vi "View.vi"(0 "object in":refnum<class "DataType.lvclass">, 2 "Requirements":T2, 5 "error in (no error)":errorcluster) -> (14 "object out":refnum<class "DataType.lvclass">, 16 "Message":T1, 19 "error out":errorcluster)   [LabVIEW 2024, in "DataType.lvclass"]
uses:
  DataType.lvclass
  Support/Type Def/Requirements.ctl
  Support/Type Def/File Type.ctl
  Support/Type Def/Message.ctl
  DataType.lvclass/DataType.ctl
panel:
  # "Connector Pane"
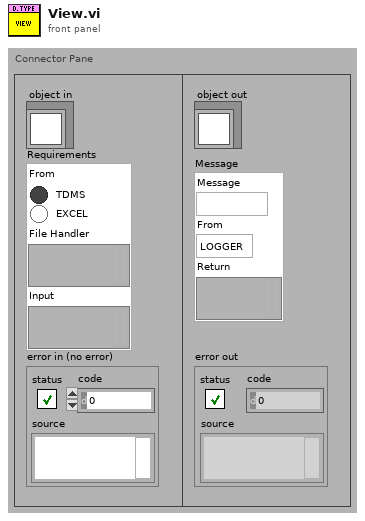
[diagram p1: front panel]
types:
  T1 = typedef "Message.ctl" = cluster{"Message":string, "From":enum16{"LOGGER", "VIEWER"}, "Return":variant}
  T2 = typedef "Requirements.ctl" = cluster{"From":T3, "File Handler":variant, "Input":variant}
  T3 = typedef "File Type.ctl" = enum32{"TDMS", "EXCEL"}
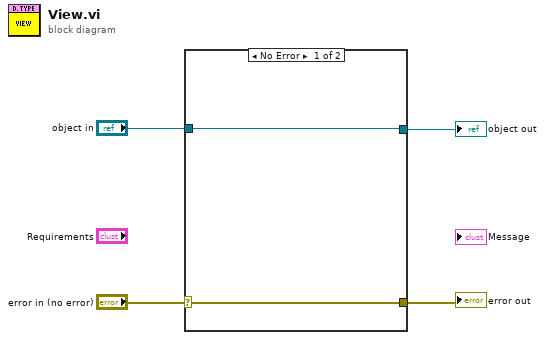
[diagram p0: block diagram]
diagram:
  n1 = case shown="No Error" "error in (no error)" {
    selector: "error in (no error)" -> [w6 w8]
    tunnel: [w6 w8] -> w3
    tunnel: [w5 w7] -> w1
    tunnel: "object in" -> [w5 w7]
    frame No Error {
    }
    frame Error {
    }
  }
  "error out" <- w3
  "object out" <- w1
